vi "Send Single Message To Specific Target.vi"(8 "error in (no error)":errorcluster, 9 "Mail Strategy In":refnum<class "Mail Strategy.lvclass">, 10 "Message In":refnum<class "Message.lvclass">, 11 "Messenger in":refnum<class "Tree-ArrayLocation Queue Messenger.lvclass">) -> (0 "error out":errorcluster, 3 "Messenger out":refnum<class "Tree-ArrayLocation Queue Messenger.lvclass">)   [LabVIEW 2019, in "Tree-ArrayLocation Queue Messenger.lvclass"]
uses:
  Tree-ArrayLocation Queue Messenger.lvclass
  C:/Users/iio/Desktop/NTHU Brain Center/General Purpose/Classes/Ancestor/Messenger/Messenger Composite/Messenger Composite.lvclass
  Ancestor Class/Messenger/Mail Strategy/Mail Strategy.lvclass
  Ancestor Class/Message/Message.lvclass
  Array Location Mailman/Array Location Mailman.lvclass
  C:/Users/iio/Desktop/NTHU Brain Center/General Purpose/Classes/Ancestor/Messenger/Mail Strategy/Mail Strategy.lvclass
  Array Location Mailman/Array Location Mailman.lvclass/Array Location Mailman.ctl
  Ancestor Class/Messenger/Messenger Composite/Messenger Composite.lvclass/Messenger Composite.ctl
  Tree-ArrayLocation Queue Messenger.lvclass/Tree-ArrayLocation Queue Messenger.ctl
  Array Location Mailman/Public Data/Write Location.vi
  Ancestor Class/Messenger/Messenger Composite/Public Data/Read Nodes.vi
  Array Location Mailman/Public Data/Read Location.vi
  Ancestor Class/Messenger/Messenger/Messenger.lvclass
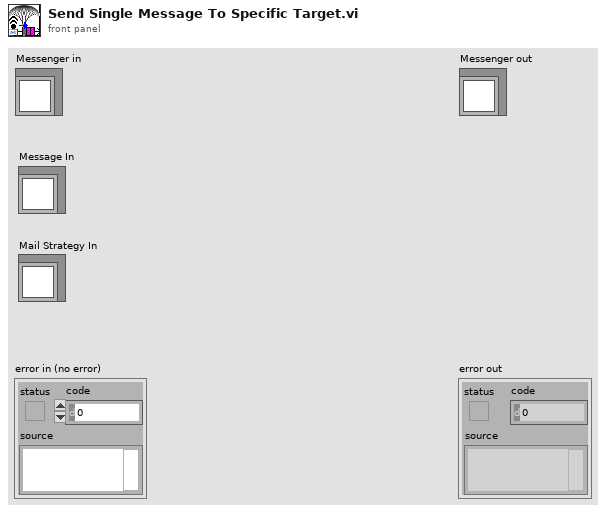
[diagram p1: front panel]
types:
  T1 = typedef "Message Queue.ctl" = refnum<queue>
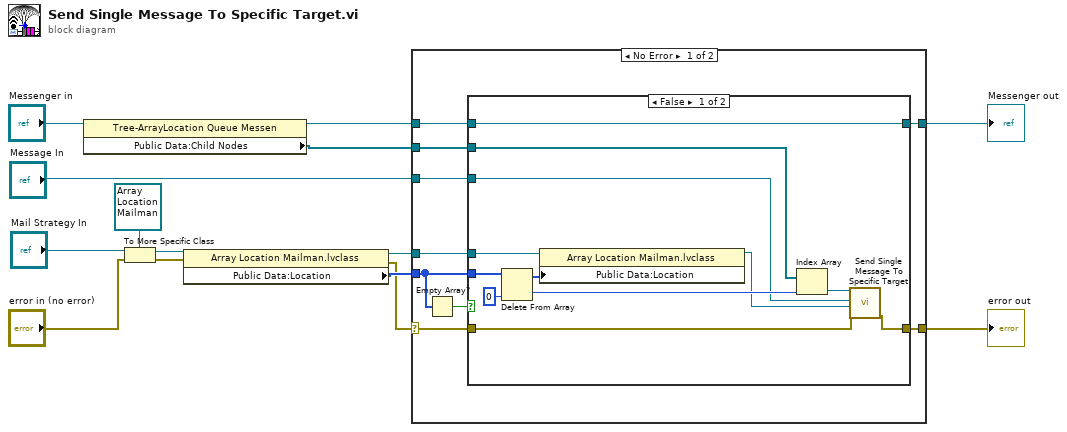
[diagram p0: block diagram]
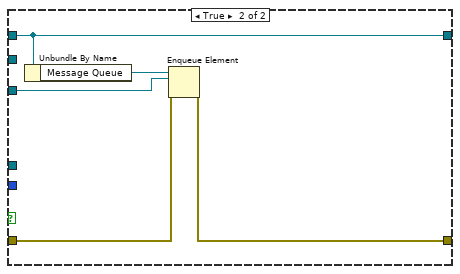
[diagram p2: hidden frame]
diagram:
  n1 = property class="Tree-ArrayLocation Queue Messen"(reference="Messenger in") -> (reference out=w4:refnum<class "Tree-ArrayLocation Queue Messenger.lvclass">, "Public Data:Child Nodes"=w3:refnum<class "Messenger.lvclass">[])  [unwired: 1 in, 1 out]
  n2 = To More Specific Class(target class=refnum<class "Array Location Mailman.lvclass"> refnum ("Array Location Mailman.lvclass"), reference="Mail Strategy In", error in="error in (no error)") -> (specific class reference=w9:refnum<class "Array Location Mailman.lvclass">, error out=w10:errorcluster)
  n3 = property class="Array Location Mailman.lvclass"(reference=w9, error in=w10) -> (reference out=w2:refnum<class "Array Location Mailman.lvclass">, error out=w7:errorcluster, "Public Data:Location"=w8:i32[])
  n4 = case shown="No Error" w7 {
    selector: w7 -> [w18 w41]
    tunnel: w4 -> [w22 w42]
    tunnel: [w20 w42] -> w14
    tunnel: [w17 w41] -> w13
    tunnel: w8 -> [w19 _]
    tunnel: "Message In" -> [w21 _]
    tunnel: w3 -> [w16 _]
    tunnel: w2 -> [w15 _]
    frame No Error {
      n5 = Empty Array?(array=w19) -> (empty?=w23:bool)
      n6 = case shown="False" w23 {
        tunnel: w22 -> [w35 w40]
        tunnel: w21 -> [w27 w38]
        tunnel: [w35 w40] -> w20
        tunnel: w19 -> [w34 _]
        tunnel: w18 -> [w25 w37]
        tunnel: [w24 w36] -> w17
        tunnel: w16 -> [w31 _]
        tunnel: w15 -> [w30 _]
        frame False {
          n7 = Delete From Array(array=w34, index=0) -> (deleted portion=w32:i32, array with subset deleted=w29:i32[])  [unwired: 1 in]
          n8 = property class="Array Location Mailman.lvclass"(reference=w30, "Public Data:Location"=w29) -> (reference out=w26:refnum<class "Array Location Mailman.lvclass">)  [unwired: 1 in, 1 out]
          n9 = Index Array(array=w31, index=w32) -> (element=w28:refnum<class "Messenger.lvclass">)
          n10 = call-dynamic "Send Single Message To Specific Target.vi"("error in (no error)"=w25, "Mail Strategy In"=w26, "Message In"=w27, "Messenger in"=w28) -> ("error out"=w24:errorcluster)  [unwired: 6 in, 1 out]
        }
        frame True {
          n11 = Unbundle By Name(w40) -> ("Message Queue"=w39:T1)
          n12 = Enqueue Element(queue=w39, element=w38, error in (no error)=w37) -> (error out=w36:errorcluster)  [unwired: 1 in, 2 out]
        }
      }
    }
    frame Error {
    }
  }
  "error out" <- w13
  "Messenger out" <- w14
